vi "test_Add Response_Variable Duplicate Error.vi"(8 "error in (no error)":errorcluster, 11 "TestCase in":refnum<class "Instrument Addon Scripting API Messages Unit Tests.lvclass">) -> (0 "error out":errorcluster, 3 "TestCase out":refnum<class "Instrument Addon Scripting API Messages Unit Tests.lvclass">)   [LabVIEW 2018, in "Instrument Addon Scripting API Messages Unit Tests.lvclass"]
uses:
  Instrument Addon Scripting API Messages Unit Tests.lvclass
  APIs/Scripting API/TypeDefs/Linked Channel.ctl
  <vilib>/NI Veristand/Custom Device API/Custom Device Item Ref.ctl
  APIs/Scripting API/TypeDefs/Wait Response Settings.ctl
  Addon/Addon Shared/SubVIs/Constants.vi
  <vilib>/NI/NI VeriStand Advanced SysDef API/_SubVIs/SysDef.Search.GUID.vi
  APIs/Scripting API/Messages/Add Response - Wait (sec).vi
  <vilib>/addons/_JKI Toolkits/VI Tester/TestCase.llb/TestCase.lvclass
  Instrument Addon Scripting API Test Assets/Instrument Addon Scripting API Test Assets.lvclass
  APIs/Scripting API/Instrument Addon Scripting API.lvlib
  <vilib>/NI Veristand/Custom Device API/Custom Device API.lvlib
  <vilib>/NI/NI VeriStand Advanced SysDef API/SysDef API/Advanced System Definition.lvlib
  Addon/Addon Shared/Instrument Addon Shared.lvlib
  C:/Program Files (x86)/National Instruments/LabVIEW 2018/vi.lib/addons/_JKI Toolkits/VI Tester/TestCase.llb/TestCase.lvclass
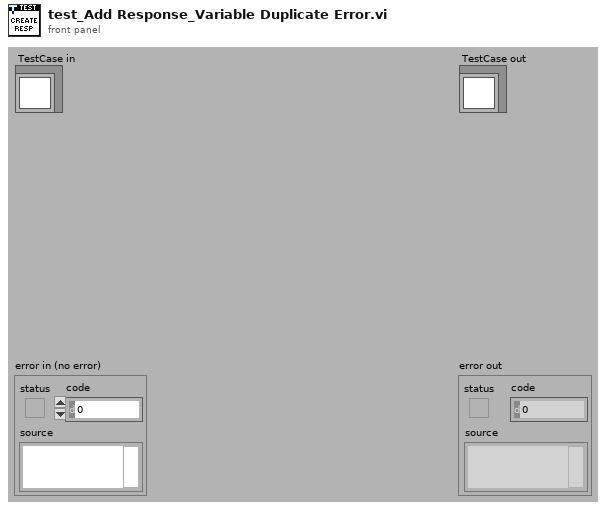
[diagram p1: front panel]
types:
  T1 = typedef "Instrument Addon Scripting API.lvlib/Wait Response Settings.ctl" = cluster{"Response Format":string, "Linked Channels":T2[], "Wait value (sec)":dbl, "Use Byte Count channel":bool, "Channel Refnum":T3}
  T2 = typedef "Instrument Addon Scripting API.lvlib/Linked Channel.ctl" = cluster{"Variable Name":string, "Channel Refnum":T3}
  T3 = typedef "Custom Device API.lvlib/Custom Device Item Ref.ctl" = u64
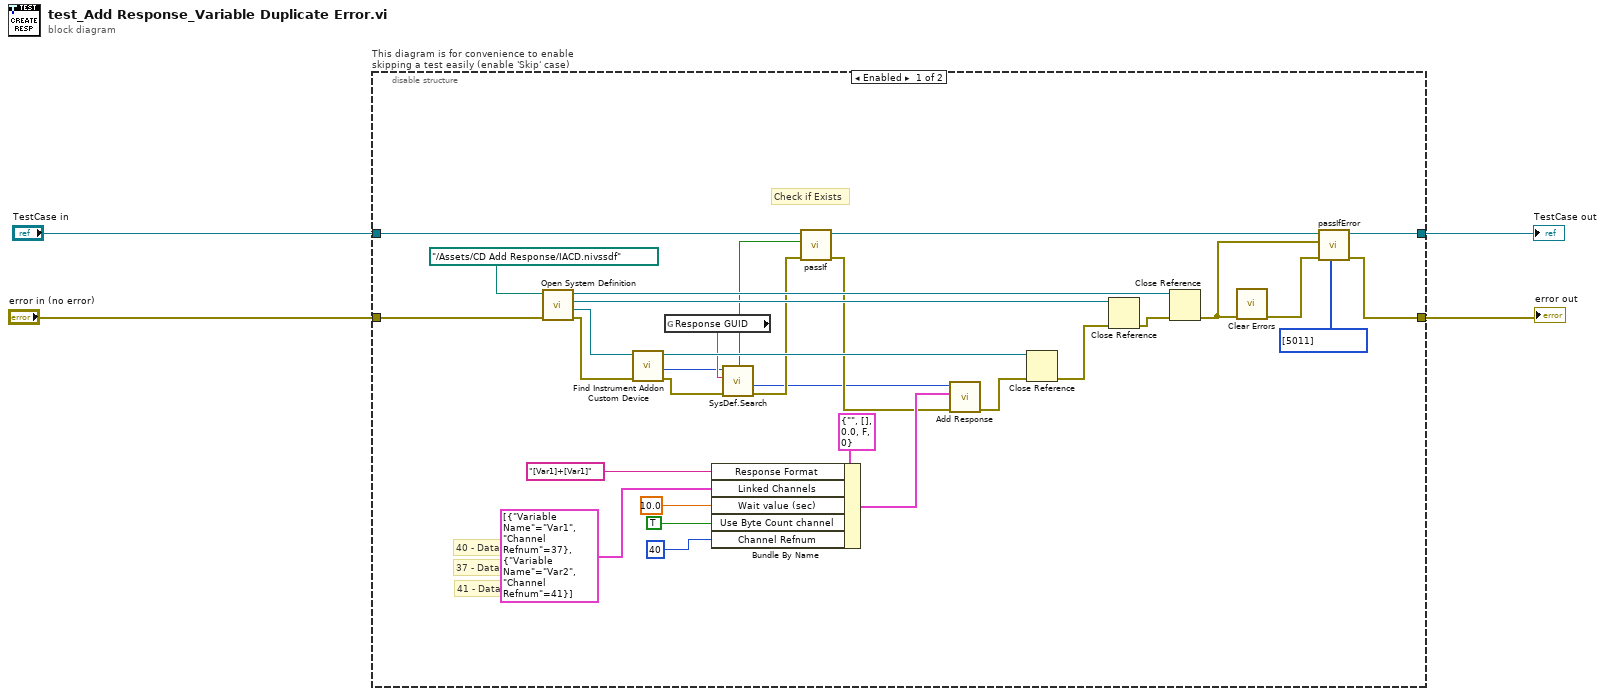
[diagram p0: block diagram]
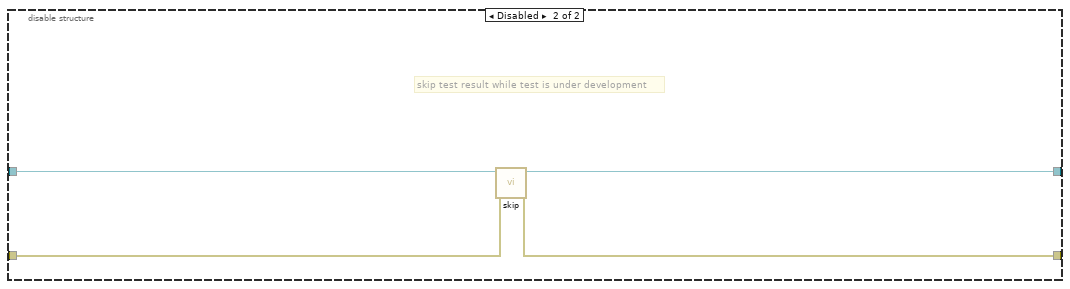
[diagram p2: hidden frame]
diagram:
  n1 = disable-structure "This diagram is for convenience to enable skipping a test easily (enable 'Skip' case)" shown="Enabled" {
    disable-tunnel: "TestCase in" -> [w19 w39]
    disable-tunnel: [w10 w37] -> w1
    disable-tunnel: [w9 w38] -> w3
    disable-tunnel: "error in (no error)" -> [w34 w36]
    frame Enabled {
      # "Check if Exists"
      # "41 - Data 2"
      # "40 - Data 0"
      # "37 - Data 1"
      n2 = call "Open System Definition.vi"("error in (no error)"=w34, "System Definition File"=path "../Assets/CD Add Response/IACD.nivssdf" ("SDF file")) -> ("error out"=w32:errorcluster, "Target Refnum"=w31:refnum<k24>, "Root Refnum"=w30:refnum<k24>, "System Definition Refnum"=w24:refnum<k24>)  [unwired: 6 in]
      n3 = call "Find Instrument Addon Custom Device.vi"("error in"=w32, "target in"=w31) -> ("error out"=w21:errorcluster, "NodeID"=w20:u64, "target out"=w29:refnum<k24>)  [unwired: 7 in]
      n4 = global read "Constants.vi" "Response GUID"() -> (w22:string)
      n5 = Bundle By Name(cluster=T1 {"Response Format"="", "Linked Channels"=[], "Wait value (sec)"=0.0, "Use Byte Count channel"=FALSE, "Channel Refnum"=0} ("Settings"), "Response Format"="[Var1]+[Var1]", "Linked Channels"=T2[] [{"Variable Name"="Var1", "Channel Refnum"=37}, {"Variable Name"="Var2", "Channel Refnum"=41}], "Wait value (sec)"=10.0, "Use Byte Count channel"=TRUE, "Channel Refnum"=T3 40) -> (w14:T1)
      n6 = call-poly <vilib>:"SysDef.Search.vi"("error in (no error)"=w21, "GUID"=w22, "nodeID"=w20) -> ("error out"=w17:errorcluster, "Value out"=w5:u64, "Found?"=w18:bool)  [unwired: 5 in, 1 out]
      n7 = call-dynamic "passIf.vi"("error in (no error)"=w17, "pass"=w18, "TestCase in"=w19) -> ("error out"=w12:errorcluster, "TestCase out"=w11:refnum<class "Instrument Addon Scripting API Messages Unit Tests.lvclass">)  [unwired: 7 in]
      n8 = call-poly "Add Response.vi"("error in (no error)"=w12, "Settings"=w14, "Message in"=w5) -> ("error out"=w13:errorcluster)  [unwired: 7 in, 1 out]
      n9 = Close Reference(reference=w29, error in (no error)=w13) -> (error out=w33:errorcluster)
      n10 = Close Reference(reference=w30, error in (no error)=w33) -> (error out=w23:errorcluster)
      n11 = Close Reference(reference=w24, error in (no error)=w23) -> (error out=w7:errorcluster)
      n12 = call <vilib>:"Clear Errors.vi"("error in (no error)"=w7) -> ("error out"=w6:errorcluster)  [unwired: 5 in, 1 out]
      n13 = call-dynamic "passIfError.vi"("passing error codes (default = any error code)"=i32[] [5011], "error in (no error)"=w6, "error"=w7, "TestCase in"=w11) -> ("error out"=w9:errorcluster, "TestCase out"=w10:refnum<class "Instrument Addon Scripting API Messages Unit Tests.lvclass">)  [unwired: 6 in]
    }
    frame Disabled {
      # "skip test result while test is under development"
      n14 = call <vilib>:"skip.vi"("error in (no error)"=w36, "TestCase in"=w39) -> ("error out"=w38:errorcluster, "TestCase out"=w37:refnum<class "Instrument Addon Scripting API Messages Unit Tests.lvclass">)  [unwired: 8 in]
    }
  }
  "error out" <- w3
  "TestCase out" <- w1
